vi "Easy Fixed-Point Filter Modeling and Simulation.vi"() -> ()   [LabVIEW 2023]
doc: "Demonstrates how to use the DFD FXP Quantize Coef VI to quantize the coefficients of a floating-point filter, and how to use the DFD FXP Modeling VI to create a fixed-point model for the quantized filter by specifying only the input and output word lengths.\n\nComplete the following steps to use this VI.\n1) Run the VI.\n2) Change the settings of the signal and the word length values, such as the <B>Source</B>, <B>Number of Samples</B>, <B>Input Word Length</B>, and <B>Output Word Length</B>.\n3) Observe the mean squared error (MSE) value and the Filtered Signals graph to understand how your changes affect the filtering result.\n4) Click the <B>STOP</B> button to stop this VI."
uses:
  <vilib>/addons/Digital Filter Design/_Objects.llb/DFD Quantization Sources.ctl
  <vilib>/addons/Digital Filter Design/FXPModel.llb/DFD FXP Quantize Coef (Easy).vi
  <vilib>/addons/Digital Filter Design/FXPModel.llb/DFD FXP Get Quantizer (One).vi
  <vilib>/Utility/VariantDataType/GetNumericFxpInfo.vi
  <vilib>/addons/Digital Filter Design/FXPSim.llb/dfd_Check Input FXP Settings.vi
  <vilib>/addons/Digital Filter Design/FXPSim.llb/dfd_Check SRate Simulation Integer Input.vi
  <vilib>/addons/Digital Filter Design/FXPSim.llb/dfd_FXP Simu.vi
  <vilib>/addons/Digital Filter Design/Process.llb/DFD Filtering (Array).vi
  <vilib>/addons/Digital Filter Design/_Objects.llb/DFD FXP Statistics Data.ctl
  <vilib>/addons/Digital Filter Design/FXPSim.llb/SimXnode/DFD FXP Simulation.xnode
  <vilib>/addons/Digital Filter Design/_Objects.llb/DFD Filter Obj.ctl
  <vilib>/addons/Digital Filter Design/_Objects.llb/DFD Filter Coef.ctl
  <vilib>/addons/Digital Filter Design/_Objects.llb/DFD Filter Structure Type Selector.ctl
  <vilib>/addons/Digital Filter Design/_Objects.llb/dfd_Internal Quantization Settings.ctl
  <vilib>/addons/Digital Filter Design/_Objects.llb/dfd_Internal Quantization Srcs.ctl
  <vilib>/addons/Digital Filter Design/_Objects.llb/DFD Coef Norm Type.ctl
  <vilib>/Analysis/NI_AALBase.lvlib
  <vilib>/addons/Digital Filter Design/NI_DigFilterLicensed.lvlib
  <vilib>/Analysis/NI_AALPro.lvlib
  <vilib>/addons/Digital Filter Design/NI_DigFilter_FXP.lvlib
  <vilib>/Utility/VariantDataType/VariantType.lvlib
panel:
  out "MSE":dbl format="%.6g"
  in  "Output Word Length":i16=16 min=1 max=32
  in  "Input Word Length":i16=16 min=1 max=32
  in  "Source":enum16{"Sine", "Random Noise"}(ring)
  in  "Number of Samples":i32=128
  in  "stop":bool
  out "Filtered Signals":dbl[][](graph)
  # "Select Help>>Show Context Help and move the cursor over the VI icon for more information."
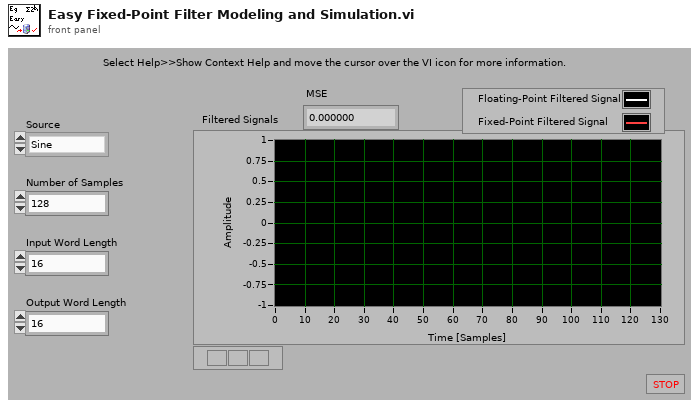
[diagram p1: front panel]
types:
  T1 = typedef "NI_DigFilterLicensed.lvlib/DFD Filter Obj.ctl" = cluster{"mSRate_Fs":dbl, "mSRate_Version":string, "mSRate_Comments":string, "mSRate_OrgCoef":T2, "mSRate_CurCoef":T2, "mSRate_Quantized?":bool, "mSRate_QCoef":T2, "mSRate_QSettings":T4[], "mSRate_Order":i32, "mSRate_Scaling":cluster{"mSRate_ScaleByPowerOf2?":bool, "mSRate_ScaleType":T6}}
  T2 = typedef "NI_DigFilterLicensed.lvlib/DFD Filter Coef.ctl" = cluster{"type":T3, "gain":dbl, "coef a (k)":dbl[], "coef b (v)":dbl[]}
  T3 = typedef "NI_DigFilterLicensed.lvlib/DFD Filter Structure Type Selector.ctl" = enum16{"Undefined", "FIR Direct Form", "FIR Direct Form Transposed", "FIR Symmetric", "FIR Antisymmetric", "IIR Direct Form I", "IIR Direct Form I Transposed", "IIR Direct Form II", "IIR Direct Form II Transposed", "IIR Cascaded Second Order Sections Form I", "IIR Cascaded Second Order Sections Form I Transposed", "IIR Cascaded Second Order Sections Form II", "IIR Cascaded Second Order Sections Form II Transposed", "Lattice Allpass (basic sections)", "Lattice Allpass (one multiplier sections)", "Lattice Allpass (normalized sections)", "Lattice AR (basic sections)", "Lattice AR (one multiplier sections)", "Lattice AR (normalized sections)", "Lattice MA (minimum phase)", "Lattice MA (maximum phase)", "Lattice ARMA (basic sections)", "Lattice ARMA (one multiplier sections)", "Lattice ARMA (normalized sections)"}
  T4 = typedef "NI_DigFilterLicensed.lvlib/dfd_Internal Quantization Settings.ctl" = cluster{"source":T5, "wl":i16, "iwl":i16, "overflow mode":enum16{"Saturation", "Wrap"}, "rounding mode":enum16{"Nearest", "Truncation"}, "signed?":bool}
  T5 = typedef "NI_DigFilterLicensed.lvlib/dfd_Internal Quantization Srcs.ctl" = u16
  T6 = typedef "NI_DigFilterLicensed.lvlib/DFD Coef Norm Type.ctl" = enum16{"No Norm", "Time Domain 1-Norm", "Time Domain 2-Norm", "Time Domain Inf-Norm"}
  T7 = typedef "NI_DigFilterLicensed.lvlib/DFD Quantization Sources.ctl" = u16
  T8 = typedef "NI_DigFilterLicensed.lvlib/DFD Quantization Settings.ctl" = cluster{"source":T7, "wl":i16, "iwl":i16, "overflow mode":enum16{"Saturation", "Wrap"}, "rounding mode":enum16{"Nearest", "Truncation"}, "signed?":bool}
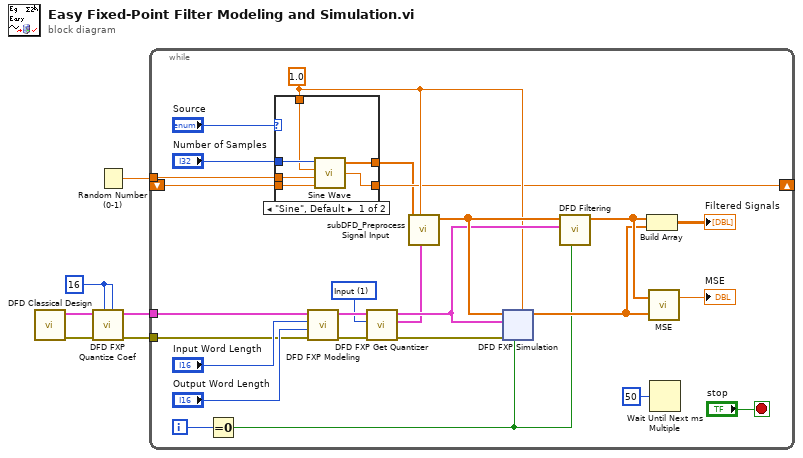
[diagram p0: block diagram]
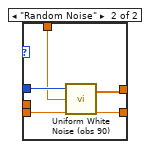
[diagram p2: hidden frame]
diagram:
  w4 = i16 16 ("coefficients a/k wl")
  n1 = call <vilib>:"DFD Classical Design.vi"() -> ("error out"=w5:errorcluster, "filter out"=w6:T1)  [unwired: 6 in, 4 out]
  n2 = call-poly <vilib>:"DFD FXP Quantize Coef.vi"("coefficients b/v word length"=w4, "coefficients a/k word length"=w4, "error in (no error)"=w5, "filter in"=w6) -> ("error out"=w3:errorcluster, "filter out"=w2:T1)  [unwired: 1 in, 5 out]
  n3 = Random Number (0-1)() -> (number: 0 to 1=w1:dbl)
  n4 = while {
    tunnel: w2 -> [w25]
    tunnel: w3 -> [w24]
    shift-right: [w9] -> _
    shift-left: _ -> [w10]
    tunnel: w1 -> [w7]
    i -> [w23]
    stop <- "stop" stop-if-true
    w12 = 1.0 ("amplitude")
    w14 = T7 1 items=["Coefficients a/k"=0, "Coefficients b/v"=7, "Input"=1, "Output"=2, "Multiplicand"=3, "Product"=4, "Sum"=5, "Delay"=6] ("quantizer source")
    n5 = Equal To 0?(x=w23) -> (x = 0?=w11:bool)
    n6 = case shown="\"Sine\", Default" "Source" {
      tunnel: [w71 w74] -> w8
      tunnel: "Number of Samples" -> [w70 w75]
      tunnel: w12 -> [w69 w73]
      tunnel: w10 -> [w68 w72]
      tunnel: [w67 w72] -> w9
      tunnel: w7 -> [w66 _]
      frame "Sine", Default {
        n7 = call <vilib>:"Sine Wave.vi"("samples"=w70, "amplitude"=w69, "frequency"=w66, "phase in"=w68) -> ("sine wave"=w71:dbl[], "phase out"=w67:dbl)  [unwired: 1 in, 1 out]
      }
      frame "Random Noise" {
        n8 = call <vilib>:"Uniform White Noise (obs 90).vi"("amplitude"=w73, "samples"=w75) -> ("uniform white noise"=w74:dbl[])  [unwired: 1 in, 1 out]
      }
    }
    n9 = call <vilib>:"DFD FXP Modeling.vi"("error in (no error)"=w24, "output word length"="Output Word Length", "input word length"="Input Word Length", "filter in"=w25) -> ("error out"=w16:errorcluster, "filter out"=w18:T1)  [unwired: 3 in, 3 out]
    n10 = call-poly <vilib>:"DFD FXP Get Quantizer.vi"("error in (no error)"=w16, "quantizer source"=w14, "filter in"=w18) -> ("error out"=w15:errorcluster, "quantizer"=w13:T8, "filter out"=w17:T1)  [unwired: 6 out]
    n11 = call <vilib>:"subDFD_Preprocess Signal Input.vi"("input quantizer"=w13, "input range"=w12, "x"=w8) -> ("q[x]"=w19:dbl[])  [unwired: 8 out]
    n12 = xnode "DFD FXP Simulation"("input range"=w12, "init? (T)"=w11, "error in (no error)"=w15, "filter in"=w17, "signal in"=w19) -> ("DBL signal out"=w21:dbl[])  [unwired: 4 out]
    n13 = call-poly <vilib>:"DFD Filtering.vi"("init? (F)"=w11, "filter"=w17, "signal in"=w19) -> ("signal out"=w22:dbl[])  [unwired: 1 in, 7 out]
    n14 = Build Array(w22, w21) -> (→"Filtered Signals":dbl[][])
    n15 = call <vilib>:"MSE.vi"("X Values"=w21, "Y Values"=w22) -> ("mse"=→"MSE":dbl)  [unwired: 1 out]
    n16 = Wait Until Next ms Multiple(millisecond multiple=u32 50) -> ()  [unwired: 1 out]
  }
